vi "Get Strings from Ref.vi"(8 "error in (no error)":errorcluster, 9 "Label Prefix":string, 10 "GObj Refnum in":refnum<vi>, 11 "Control in":refnum<class "Control.lvclass">) -> (0 "error out":errorcluster, 1 "Valid?":bool, 2 "GObj Refnum out":refnum<vi>, 3 "Control out":refnum<class "Control.lvclass">, 4 "GObj Name":string)   [LabVIEW 2013, in "SET Project Data.lvlib" / "Control.lvclass"]
uses:
  Control.lvclass
  GObject/GObject.lvclass/GObject.ctl
  GObject/Write UID.vi
  GObject/Write ClassName.vi
  GObject/Write Label.vi
  GObject/GObject.lvclass
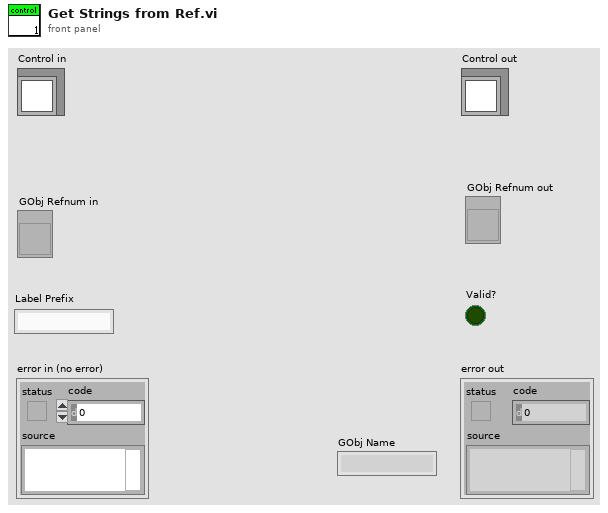
[diagram p1: front panel]
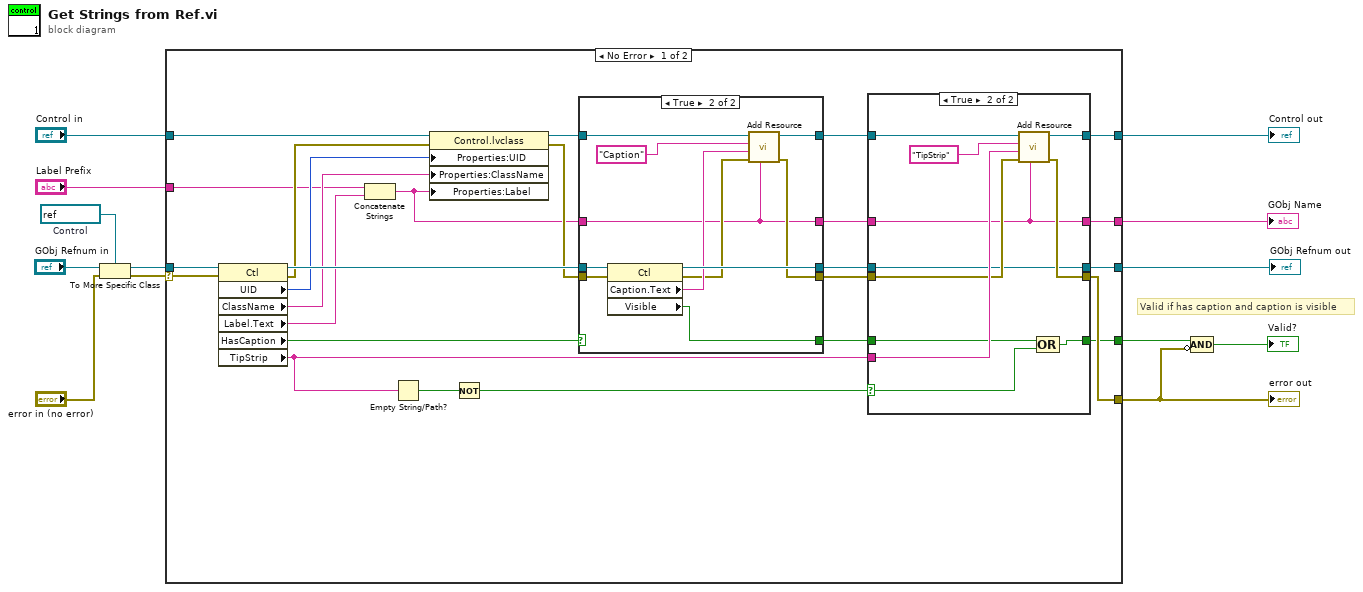
[diagram p0: block diagram]
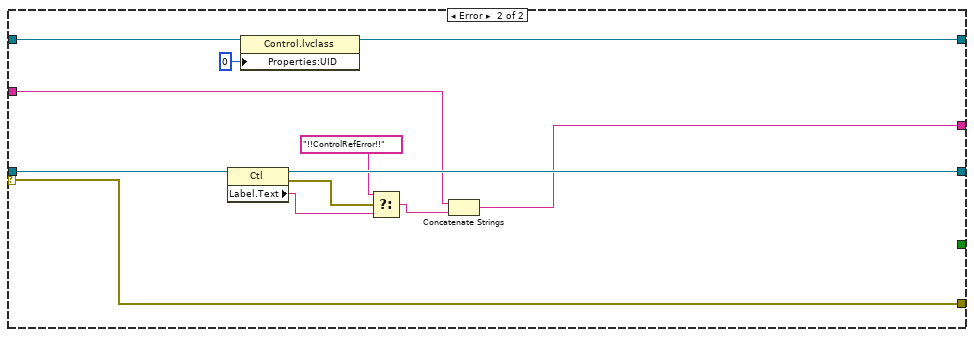
[diagram p4: hidden frame]
diagram:
  w8 = refnum<vi> refnum  # Control
  # "Valid if has caption and caption is visible"
  n1 = To More Specific Class(target class=w8, reference="GObj Refnum in", error in="error in (no error)") -> (specific class reference=w7:refnum<vi>, error out=w9:errorcluster)
  n2 = case shown="No Error" w9 {
    selector: w9 -> [w36 w83]
    tunnel: [w20 w83] -> w3
    tunnel: [w22 w80] -> w12
    tunnel: "Control in" -> [w35 w82]
    tunnel: w7 -> [w39 w79]
    tunnel: [w19 w78] -> w6
    tunnel: "Label Prefix" -> [w28 w73]
    tunnel: [w16 _] -> w4
    tunnel: [w18 w72] -> w1
    frame No Error {
      n3 = property class="Ctl"(reference=w39, error in=w36) -> (reference out=w37:refnum<vi>, error out=w31:errorcluster, "UID"=w33:i32, "ClassName"=w32:string, "Label.Text"=w29:string, "HasCaption"=w38:bool, "TipStrip"=w26:string)
      n4 = Concatenate Strings(w28, w29) -> (w27:string)
      n5 = Empty String/Path?(string/path=w26) -> (empty?=w15:bool)
      n6 = property class="Control.lvclass"(reference=w35, error in=w31, "Properties:UID"=w33, "Properties:ClassName"=w32, "Properties:Label"=w27) -> (reference out=w34:refnum<class "Control.lvclass">, error out=w30:errorcluster)
      n7 = Not(x=w15) -> (.not. x?=w14:bool)
      n8 = case shown="True" w38 {
        selector: w38 -> [w57 _]
        tunnel: w37 -> [w59 w71]
        tunnel: [w59 w70] -> w24
        tunnel: w30 -> [w60 w69]
        tunnel: [w60 w62] -> w21
        tunnel: [w58 w66] -> w23
        tunnel: w34 -> [w58 w67]
        tunnel: [w57 w68] -> w17
        tunnel: w27 -> [w56 w61]
        tunnel: [w56 w61] -> w25
        frame False {
        }
        frame True {
          n9 = property class="Ctl"(reference=w71, error in=w69) -> (reference out=w70:refnum<vi>, error out=w63:errorcluster, "Caption.Text"=w64:string, "Visible"=w68:bool)
          n10 = call "Add Resource.vi"("TagPrefix"=w61, "error in (no error)"=w63, "ItemText"=w64, "ItemName"="Caption", "GObject in"=w67) -> ("error out"=w62:errorcluster, "GObject out"=w66:refnum<class "Control.lvclass">)  [unwired: 5 in]
        }
      }
      n11 = case shown="True" w14 {
        selector: w14 -> [_ w46]
        tunnel: w26 -> [_ w52]
        tunnel: w25 -> [w41 w48]
        tunnel: w24 -> [w43 w49]
        tunnel: w23 -> [w40 w55]
        tunnel: [w40 w54] -> w22
        tunnel: w21 -> [w42 w51]
        tunnel: [w42 w50] -> w20
        tunnel: [w43 w49] -> w19
        tunnel: [w41 w48] -> w18
        tunnel: w17 -> [w44 w47]
        tunnel: [w44 w45] -> w16
        frame False {
        }
        frame True {
          n12 = call "Add Resource.vi"("TagPrefix"=w48, "error in (no error)"=w51, "ItemText"=w52, "ItemName"="TipStrip", "GObject in"=w55) -> ("error out"=w50:errorcluster, "GObject out"=w54:refnum<class "Control.lvclass">)  [unwired: 5 in]
          n13 = Compound Arithmetic op=OR(w47, w46) -> (w45:bool)
        }
      }
    }
    frame Error {
      n14 = property class="Ctl"(reference=w79) -> (reference out=w78:refnum<vi>, error out=w77:errorcluster, "Label.Text"=w75:string)  [unwired: 1 in]
      n15 = property class="Control.lvclass"(reference=w82, "Properties:UID"=0 ("UID")) -> (reference out=w80:refnum<class "Control.lvclass">)  [unwired: 1 in, 1 out]
      n16 = Select(t="!!ControlRefError!!", s=w77, f=w75) -> (s? t:f=w74:string)
      n17 = Concatenate Strings(w73, w74) -> (w72:string)
    }
  }
  "error out" <- w3
  "Control out" <- w12
  "GObj Refnum out" <- w6
  "GObj Name" <- w1
  n18 = Compound Arithmetic op=AND(w4, invert w3) -> (→"Valid?":bool)
